vi "cw_1_10.vi"() -> ()   [LabVIEW 2022 SP3]
panel:
  out "X2":cdb
  out "X1":cdb
  out "delta":dbl
  in  "C":dbl
  in  "B":dbl
  in  "A":dbl
  # "y(x) = Ax^2+Bx+C"
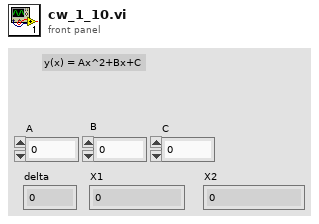
[diagram p1: front panel]
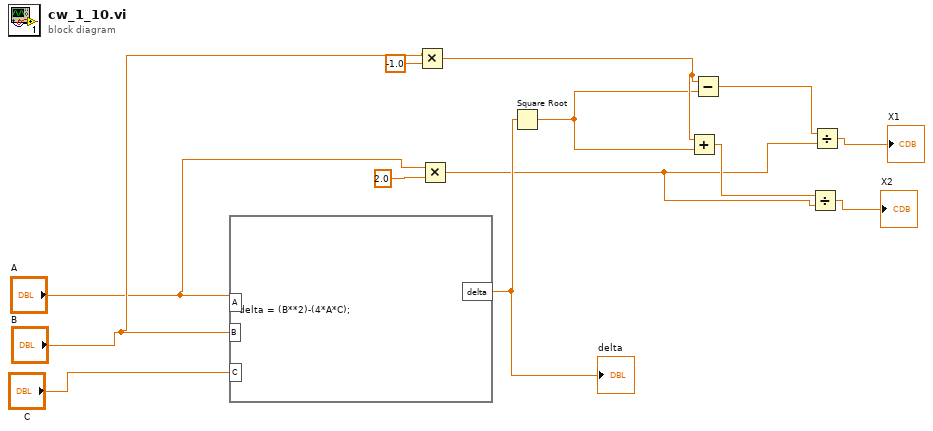
[diagram p0: block diagram]
diagram:
  n1 = formula code="delta = (B**2)-(4*A*C);"("C"="C", "B"="B", "A"="A") -> ("delta"=w12:dbl)
  "delta" <- w12
  n2 = Multiply(x="B", y=-1.0) -> (x*y=w9:dbl)
  n3 = Multiply(x="A", y=2.0) -> (x*y=w2:dbl)
  n4 = Square Root(x=w12) -> (sqrt(x)=w8:cdb)
  n5 = Add(x=w9, y=w8) -> (x+y=w3:cdb)
  n6 = Subtract(x=w9, y=w8) -> (x-y=w5:cdb)
  n7 = Divide(x=w3, y=w2) -> (x/y=→"X2":cdb)
  n8 = Divide(x=w5, y=w2) -> (x/y=→"X1":cdb)
